vi "MTM2_getNextSample_zenithAngle.vi"(8 "error in (no error)":errorcluster, 11 "zenithAngle_Ctl":T1) -> (0 "error out":errorcluster, 2 "function return":i32, 3 "zenithAngle_Ctl out":T1)   [LabVIEW 2018, in "SALLV_MTM2.lvlib"]
doc: "int MTM2_shm_getNextSample_zenithAngleLV(MTM2_zenithAngleLV *zenithAngle_Ctl );"
uses:
  DataTypes/zenithAngle.ctl
  SALLV_MTM2.lvlib
  SALLV_MTM2.so
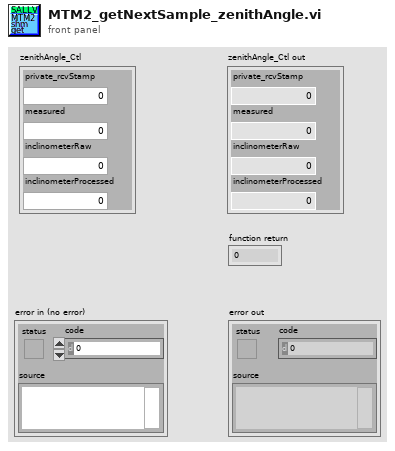
[diagram p1: front panel]
types:
  T1 = typedef "SALLV_MTM2.lvlib/zenithAngle.ctl" = cluster{"private_rcvStamp":dbl, "measured":dbl, "inclinometerRaw":dbl, "inclinometerProcessed":dbl}
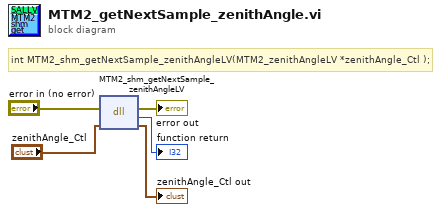
[diagram p0: block diagram]
diagram:
  # "int MTM2_shm_getNextSample_zenithAngleLV(MTM2_zenithAngleLV *zenithAngle_Ctl );"
  n1 = dll-call lib="home/ttsai/Documents/salLabviewApi/SALLV_MTM2/SALLV_MTM2.*" fn="MTM2_shm_getNextSample_zenithAngleLV"(error in="error in (no error)", "zenithAngle_Ctl"="zenithAngle_Ctl") -> (error out=→"error out":errorcluster, →"function return":i32, "zenithAngle_Ctl"=→"zenithAngle_Ctl out":T1)  [unwired: 2 in, 1 out]
